vi "MultiListBoxDuplicatesCheck.vi"(3 "CAN Init Ref In":refnum<vi>, 5 "_Write Table In":refnum<vi>, 7 "_Read Table Ref In":refnum<vi>, 8 "CAN Write Signals String Array":string[](array[string]), 11 "Flex Control Parameters String Array":string[](array[string])) -> ()   [LabVIEW 2015, in "ECS-Host.lvlib"]
uses:
  ECS-Host.lvlib
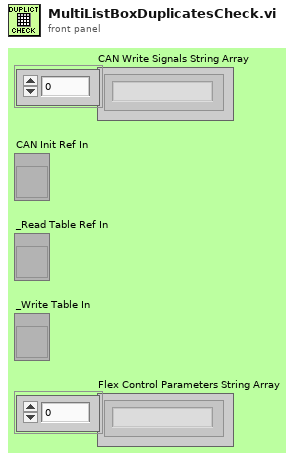
[diagram p1: front panel]
types:
  T1 = enum8{"Enabled", "Disabled", "Disabled and Grayed Out"}
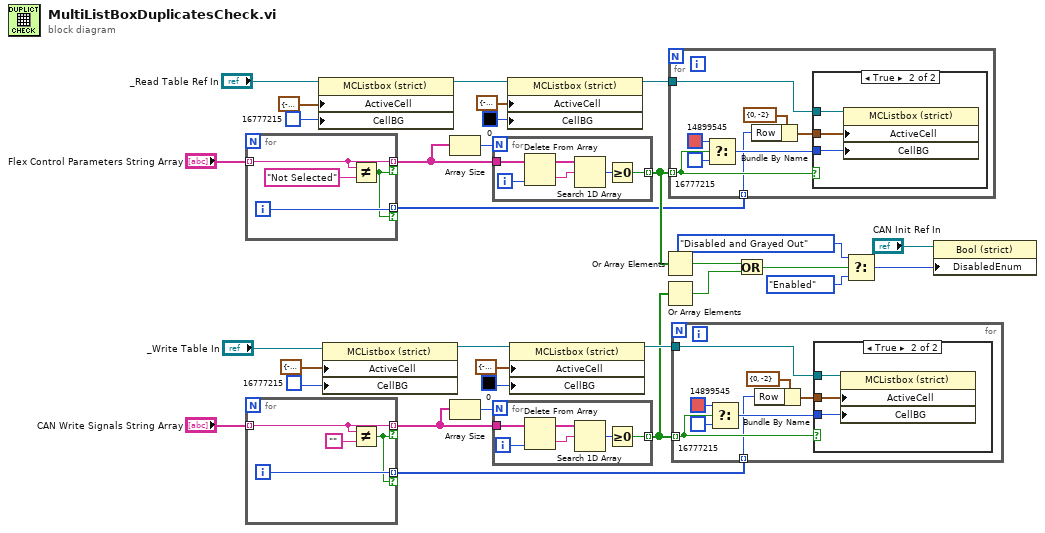
[diagram p0: block diagram]
diagram:
  n1 = for {
    tunnel: [w35] -> w4 mode=indexing if=w32
    tunnel: "Flex Control Parameters String Array" -> [w35] mode=indexing
    tunnel: [w33] -> w6 mode=indexing if=w32
    i -> [w33]
    n2 = Not Equal?(x=w35, y="Not Selected") -> (x != y?=w32:bool)
  }
  n3 = for {
    tunnel: [w39] -> w1 mode=indexing if=w36
    tunnel: "CAN Write Signals String Array" -> [w39] mode=indexing
    tunnel: [w37] -> w5 mode=indexing if=w36
    i -> [w37]
    n4 = Not Equal?(x=w39, y="") -> (x != y?=w36:bool)
  }
  n5 = property on="Property Node" class="MCListbox (strict)"(reference="_Read Table Ref In", "ActiveCell"=cluster{"Row":i32, "Column":i32} {"Row"=-2, "Column"=-2} ("Active Cell:Active Cell"), "CellBG"=u32 16777215 ("Color Box")) -> (reference out=w25:refnum<vi>)  [unwired: 1 in, 1 out]
  n6 = property on="Property Node" class="MCListbox (strict)"(reference="_Write Table In", "ActiveCell"=cluster{"Row":i32, "Column":i32} {"Row"=-2, "Column"=-2} ("Active Cell:Active Cell"), "CellBG"=u32 16777215 ("Color Box")) -> (reference out=w26:refnum<vi>)  [unwired: 1 in, 1 out]
  n7 = Array Size(array=w4) -> (size(s)=w3:i32)
  n8 = Array Size(array=w1) -> (size(s)=w2:i32)
  n9 = for {
    N: w3 -> [_]
    tunnel: w4 -> [w44]
    tunnel: [w41] -> w15 mode=indexing
    i -> [w40]
    n10 = Delete From Array(array=w44, index=w40) -> (deleted portion=w42:string, array with subset deleted=w43:string[])  [unwired: 1 in]
    n11 = Search 1D Array(1D array=w43, element=w42) -> (index of element=w45:i32)  [unwired: 1 in]
    n12 = Greater Or Equal To 0?(x=w45) -> (x >= 0?=w41:bool)
  }
  n13 = for {
    N: w2 -> [_]
    tunnel: w1 -> [w50]
    tunnel: [w47] -> w16 mode=indexing
    i -> [w46]
    n14 = Delete From Array(array=w50, index=w46) -> (deleted portion=w48:string, array with subset deleted=w49:string[])  [unwired: 1 in]
    n15 = Search 1D Array(1D array=w49, element=w48) -> (index of element=w51:i32)  [unwired: 1 in]
    n16 = Greater Or Equal To 0?(x=w51) -> (x >= 0?=w47:bool)
  }
  n17 = property on="Property Node" class="MCListbox (strict)"(reference=w25, "ActiveCell"=cluster{"Row":i32, "Column":i32} {"Row"=-1, "Column"=-2} ("Active Cell:Active Cell"), "CellBG"=u32 0 ("Color Box")) -> (reference out=w28:refnum<vi>)  [unwired: 1 in, 1 out]
  n18 = property on="Property Node" class="MCListbox (strict)"(reference=w26, "ActiveCell"=cluster{"Row":i32, "Column":i32} {"Row"=-1, "Column"=-2} ("Active Cell:Active Cell"), "CellBG"=u32 0 ("Color Box")) -> (reference out=w27:refnum<vi>)  [unwired: 1 in, 1 out]
  n19 = Or Array Elements(Boolean array=w15) -> (logical OR=w14:bool)
  n20 = Or Array Elements(Boolean array=w16) -> (logical OR=w9:bool)
  n21 = for {
    tunnel: w15 -> [w54] mode=indexing
    tunnel: w28 -> [w53]
    tunnel: w6 -> [w52] mode=indexing
    n22 = Select(t=u32 14899545 ("Color Box"), s=w54, f=u32 16777215 ("Color Box")) -> (s? t:f=w55:u32)
    n23 = Bundle By Name(cluster=cluster{"Row":i32, "Column":i32} {"Row"=0, "Column"=-2} ("Active Cell:Active Cell"), "Row"=w52) -> (w58:cluster{"Row":i32, "Column":i32})
    n24 = case shown="True" w54 {
      tunnel: w58 -> [_ w62]
      tunnel: w55 -> [_ w61]
      tunnel: w53 -> [_ w60]
      frame False {
      }
      frame True {
        n25 = property on="Property Node" class="MCListbox (strict)"(reference=w60, "ActiveCell"=w62, "CellBG"=w61) -> ()  [unwired: 1 in, 2 out]
      }
    }
  }
  n26 = for {
    tunnel: w16 -> [w65] mode=indexing
    tunnel: w27 -> [w64]
    tunnel: w5 -> [w63] mode=indexing
    n27 = Select(t=u32 14899545 ("Color Box"), s=w65, f=u32 16777215 ("Color Box")) -> (s? t:f=w66:u32)
    n28 = Bundle By Name(cluster=cluster{"Row":i32, "Column":i32} {"Row"=0, "Column"=-2} ("Active Cell:Active Cell"), "Row"=w63) -> (w69:cluster{"Row":i32, "Column":i32})
    n29 = case shown="True" w65 {
      tunnel: w69 -> [_ w73]
      tunnel: w66 -> [_ w72]
      tunnel: w64 -> [_ w71]
      frame False {
      }
      frame True {
        n30 = property on="Property Node" class="MCListbox (strict)"(reference=w71, "ActiveCell"=w73, "CellBG"=w72) -> ()  [unwired: 1 in, 2 out]
      }
    }
  }
  n31 = Or(x=w14, y=w9) -> (x .or. y?=w13:bool)
  n32 = Select(t=T1."Disabled and Grayed Out" ("Disabled"), s=w13, f=T1."Enabled" ("Disabled")) -> (s? t:f=w11:T1)
  n33 = property on="Property Node" class="Bool (strict)"(reference="CAN Init Ref In", "DisabledEnum"=w11) -> ()  [unwired: 1 in, 2 out]
